vi "fg_download_location.vi"(8 "error in (no error)":errorcluster, 11 "path in":path) -> (0 "error out":errorcluster, 3 "path out":path)   [LabVIEW 2015, in "lv-post-installer.lvlib"]
uses:
  lv-post-installer.lvlib
  <vilib>/Utility/sysdir.llb/System Directory Type.ctl
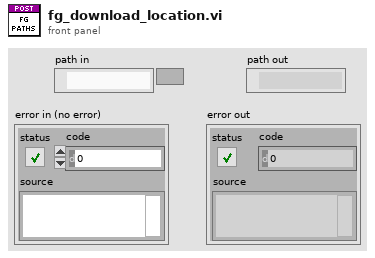
[diagram p1: front panel]
types:
  T1 = typedef "System Directory Type.ctl" = i32
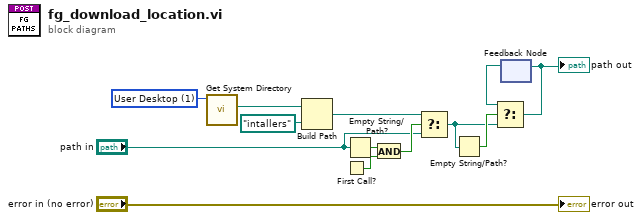
[diagram p0: block diagram]
diagram:
  w8 = T1 1 items=["User Home"=0, "User Desktop"=1, "User Documents"=2, "User Application Data"=3, "User Preferences"=4, "User Temporary"=5, "Public Documents"=6, "Public Application Data"=7, "Public Preferences"=8, "Public Cache"=13, "System Core Libraries"=9, "System Installed Libraries"=10, "Application Files"=11, "Boot Volume Root"=12] ("system directory type")
  n1 = call <vilib>:"Get System Directory.vi"("system directory type"=w8) -> ("system directory"=w7:path)  [unwired: 10 in]
  n2 = Build Path(base path=w7, name or relative path=path "intallers" ("Application Directory")) -> (appended path=w11:path)
  n3 = First Call?() -> (First Call?: T/F=w9:bool)
  n4 = Empty String/Path?(string/path="path in") -> (empty?=w5:bool)
  n5 = And(x=w5, y=w9) -> (x .and. y?=w10:bool)
  n6 = Select(t=w11, s=w10, f="path in") -> (s? t:f=w1:path)
  n7 = Empty String/Path?(string/path=w1) -> (empty?=w3:bool)
  n8 = feedback #1() -> (w2:path)  [unwired: 1 in]
  n9 = Select(t=w2, s=w3, f=w1) -> (s? t:f=w12:path)
  "path out" <- w12
  n10 = feedback-in #1(w12) -> ()
  "error out" <- "error in (no error)"
